vi "NXT parse command string.vi"(0 "String":string, 1 "error in":errorcluster) -> (2 "Remaining\nString":string, 3 "length":i32, 4 "Command":string, 5 "error out":errorcluster)   [LabVIEW 2012]
doc: "This VI parses a string sent from the PC outputing the type of command, the remaining string and its length."
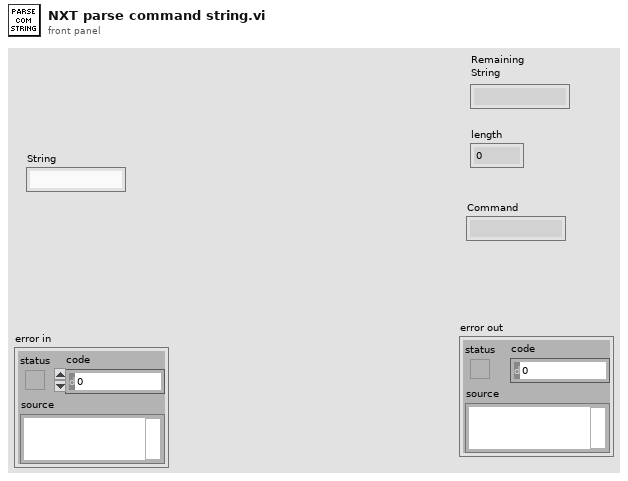
[diagram p1: front panel]
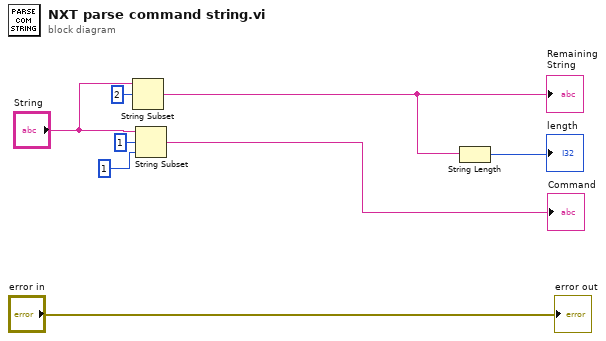
[diagram p0: block diagram]
diagram:
  n1 = String Subset(string="String", offset (0)=2) -> (substring=w2:string)  [unwired: 1 in]
  "Remaining\nString" <- w2
  n2 = String Subset(string="String", offset (0)=1, length (rest)=1 ("length (rest)")) -> (substring=→"Command":string)
  n3 = String Length(string=w2) -> (length=→"length":i32)
  "error out" <- "error in"
